vi "数据写入database.vi"(9 "data":variant, 10 "columns":string[](array[string]), 11 "table":string) -> ()   [LabVIEW 2016, in "斯坦道CODMn.lvlib"]
uses:
  <vilib>/Utility/sysdir.llb/System Directory Type.ctl
  <vilib>/addons/database/Connection.llb/DB Tools Open Connec (String).vi
  <vilib>/addons/database/NI_Database_API.lvlib
panel:
  out "error out":errorcluster
  in  "error in (no error)":errorcluster
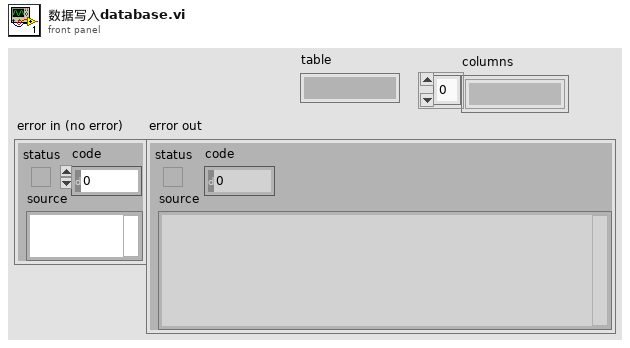
[diagram p1: front panel]
types:
  T1 = typedef "System Directory Type.ctl" = i32
  T2 = typedef "NI_Database_API.lvlib/Conn ObjectReference.ctl" = refnum<k1>
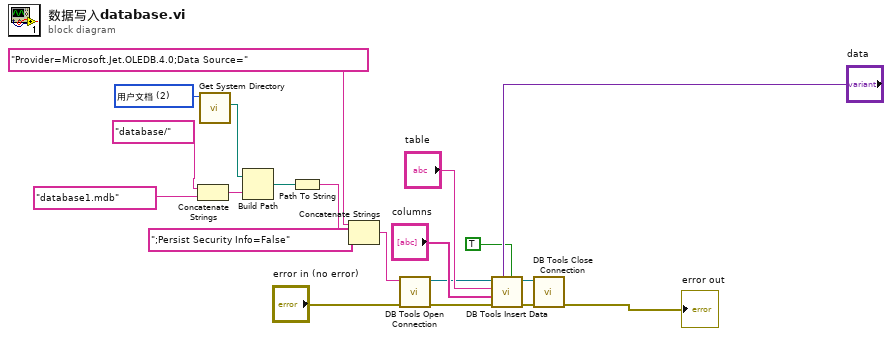
[diagram p0: block diagram]
diagram:
  w13 = T1 2 items=["用户目录"=0, "用户桌面"=1, "用户文档"=2, "用户应用程序数据"=3, "用户设置"=4, "用户临时目录"=5, "公共文档"=6, "公共应用程序数据"=7, "公共设置"=8, "公共缓存"=13, "系统核心库"=9, "系统安装库"=10, "应用程序文件"=11, "启动盘根目录"=12] ("system directory type")
  n1 = Concatenate Strings("database/" ("condition"), "database1.mdb" ("字符串")) -> (w3:string)
  n2 = call <vilib>:"Get System Directory.vi"("system directory type"=w13) -> ("system directory"=w11:path)  [unwired: 10 in]
  n3 = Build Path(base path=w11, name or relative path=w3) -> (appended path=w10:path)
  n4 = Path To String(path=w10) -> (string=w9:string)
  n5 = Concatenate Strings("Provider=Microsoft.Jet.OLEDB.4.0;Data Source=" ("condition"), w9, ";Persist Security Info=False" ("condition")) -> (w7:string)
  n6 = call-poly <vilib>:"DB Tools Open Connection.vi"("error in (no error)"="error in (no error)", "connection information"=w7) -> ("error out"=w4:errorcluster, "connection reference"=w5:T2)  [unwired: 6 in]
  n7 = call <vilib>:"DB Tools Insert Data.vi"("create table? (F)"=TRUE, "data"="data", "error in (no error)"=w4, "columns"="columns", "table"="table", "connection reference"=w5) -> ("error out"=w19:errorcluster, "connection reference out"=w20:T2)  [unwired: 4 in]
  n8 = call <vilib>:"DB Tools Close Connection.vi"("error in (no error)"=w19, "connection reference"=w20) -> ("error out"=→"error out":errorcluster)  [unwired: 5 in]
